vi "SerialRX.vi"() -> ()   [LabVIEW 2015]
uses:
  <vilib>/Instr/_visa.llb/VISA Set IO Buffer Mask.ctl
  <vilib>/Instr/_visa.llb/VISA Configure Serial Port (Instr).vi
  <vilib>/express/express analysis/Spectral/Block/exnSpectralBlock spectral measurements peak poly.vi
  <vilib>/express/express analysis/Spectral/Block/exnSpectralBlock spectral measurements peak DDT.vi
  <vilib>/express/express analysis/Spectral/XNode/ExpressSpectralMeasurementsBlockNode.xnode
  <instrlib>/Siglent SDG 1000 5000 800 Series/Siglent SDG 1000 5000 800 Series.lvlib
panel:
  in  "Boolean":bool
  out "ENOB (db)":dbl
  out "Waveform Graph 4":dbl[](graph)
  out "SINAD (dB)":dbl
  out "Waveform Graph":dynamicdata(graph)
  in  "Waveform Function (0: Sine)":u16(ring) items=["Sine", "Square", "Ramp", "DC", "Pulse", "Arb"]
  in  "Enable Output":bool
  in  "Amplitud ( Vpp )":dbl
  in  "DC Offset ( V )":dbl
  out "THD":dbl
  out "Waveform Graph 3":dynamicdata(graph)
  in  "Serial Settings":T1={"baud rate"=9600, "data bits"=8, "parity"=enum."None", "stop bits"=10, "flow control"=0} {"flow control" items=["None"=0, "XON/XOFF"=1, "RTS/CTS"=2, "DTR/DSR"=4]; "stop bits" items=["1.0"=10, "1.5"=15, "2.0"=20]; "data bits" min=5 max=8 step=1; "baud rate" items=["75"=75, "110"=110, "134"=134, "150"=150, "300"=300, "600"=600, "1200"=1200, "1800"=1800, "2400"=2400, "4800"=4800, "7200"=7200, "9600"=9600, "14400"=14400, "19200"=19200, "28800"=28800, "38400"=38400, "56000"=56000, "57600"=57600, "115200"=115200, "128000"=128000, "230400"=230400]}
  out "Waveform Graph 2":dbl[](graph)
  in  "GENERADOR":refnum<visa-resource-name>
  in  "FPGA":refnum<visa-resource-name>
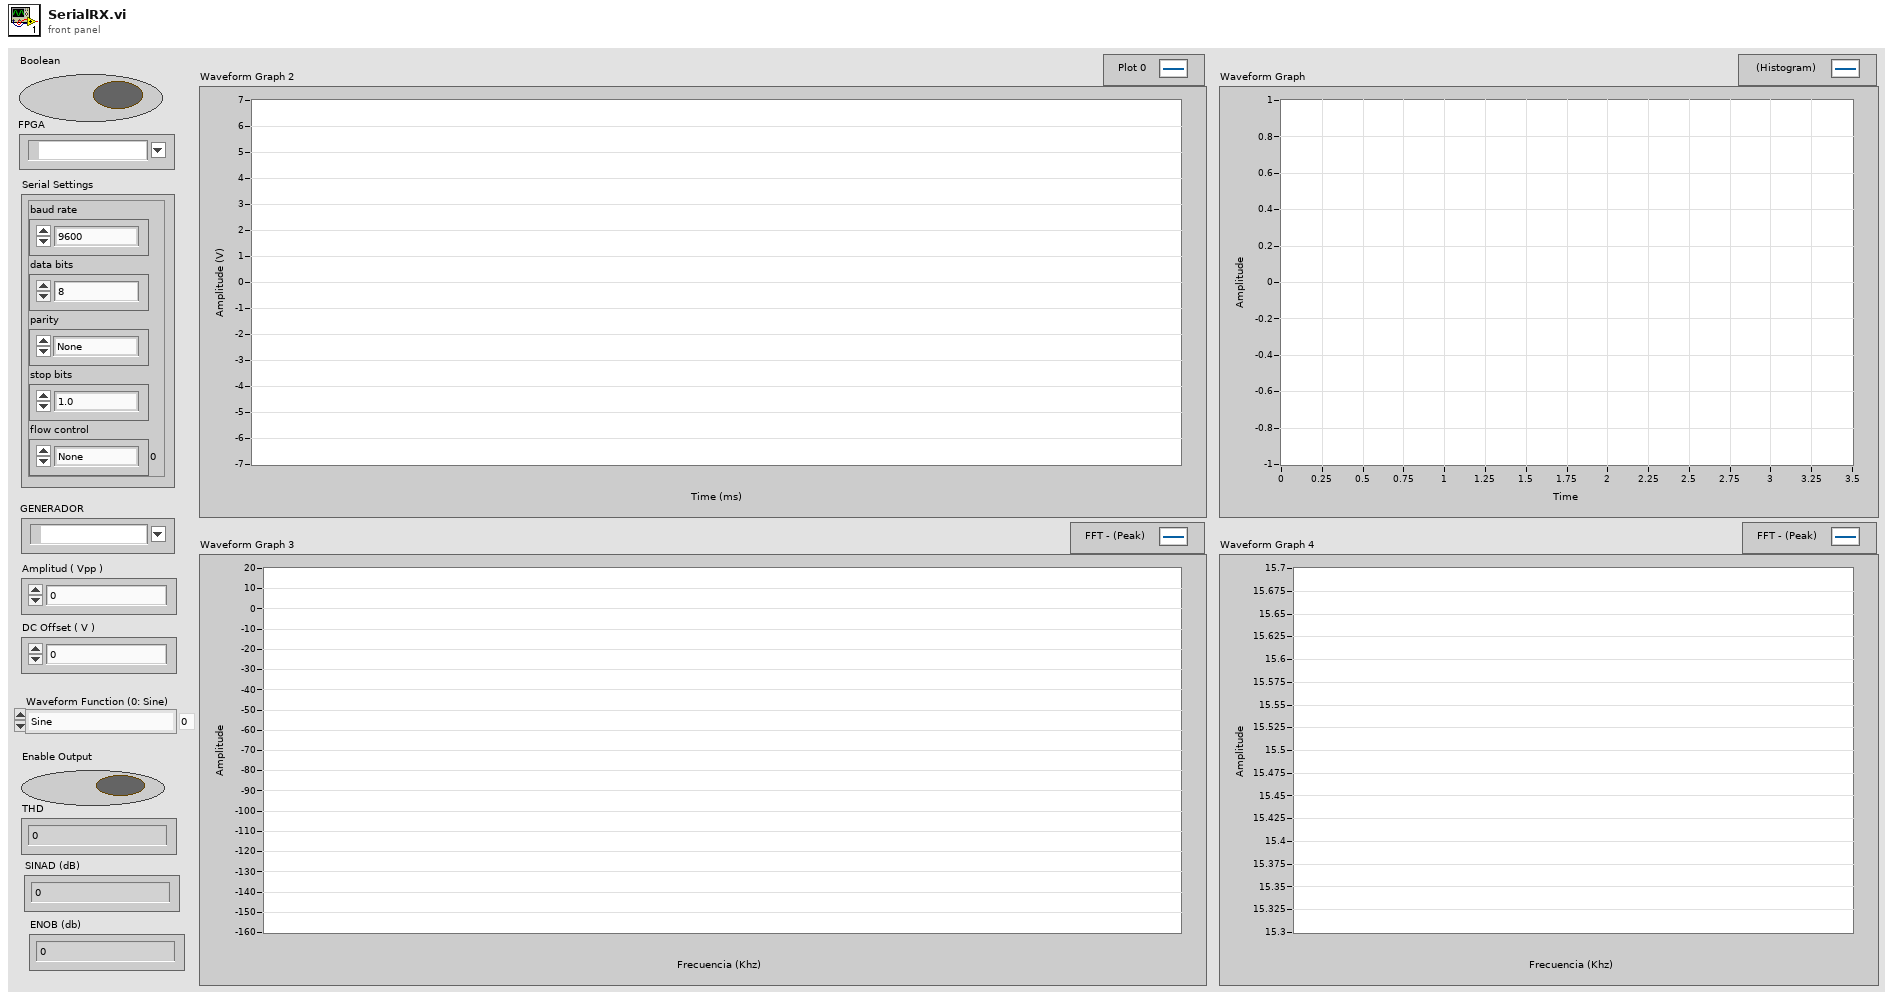
[diagram p1: front panel]
types:
  T1 = cluster{"baud rate":u32, "data bits":u16, "parity":enum16{"None", "Odd", "Even", "Mark", "Space"}, "stop bits":u16, "flow control":u16}
  T2 = typedef "VISA Set IO Buffer Mask.ctl" = u16
  T3 = cluster{"averaging mode":u16, "weighting mode":u16, "number of averages":u32}
  T4 = cluster{"dB On (F)":bool, "unwrap phase (F)":bool, "convert to degree (F)":bool}
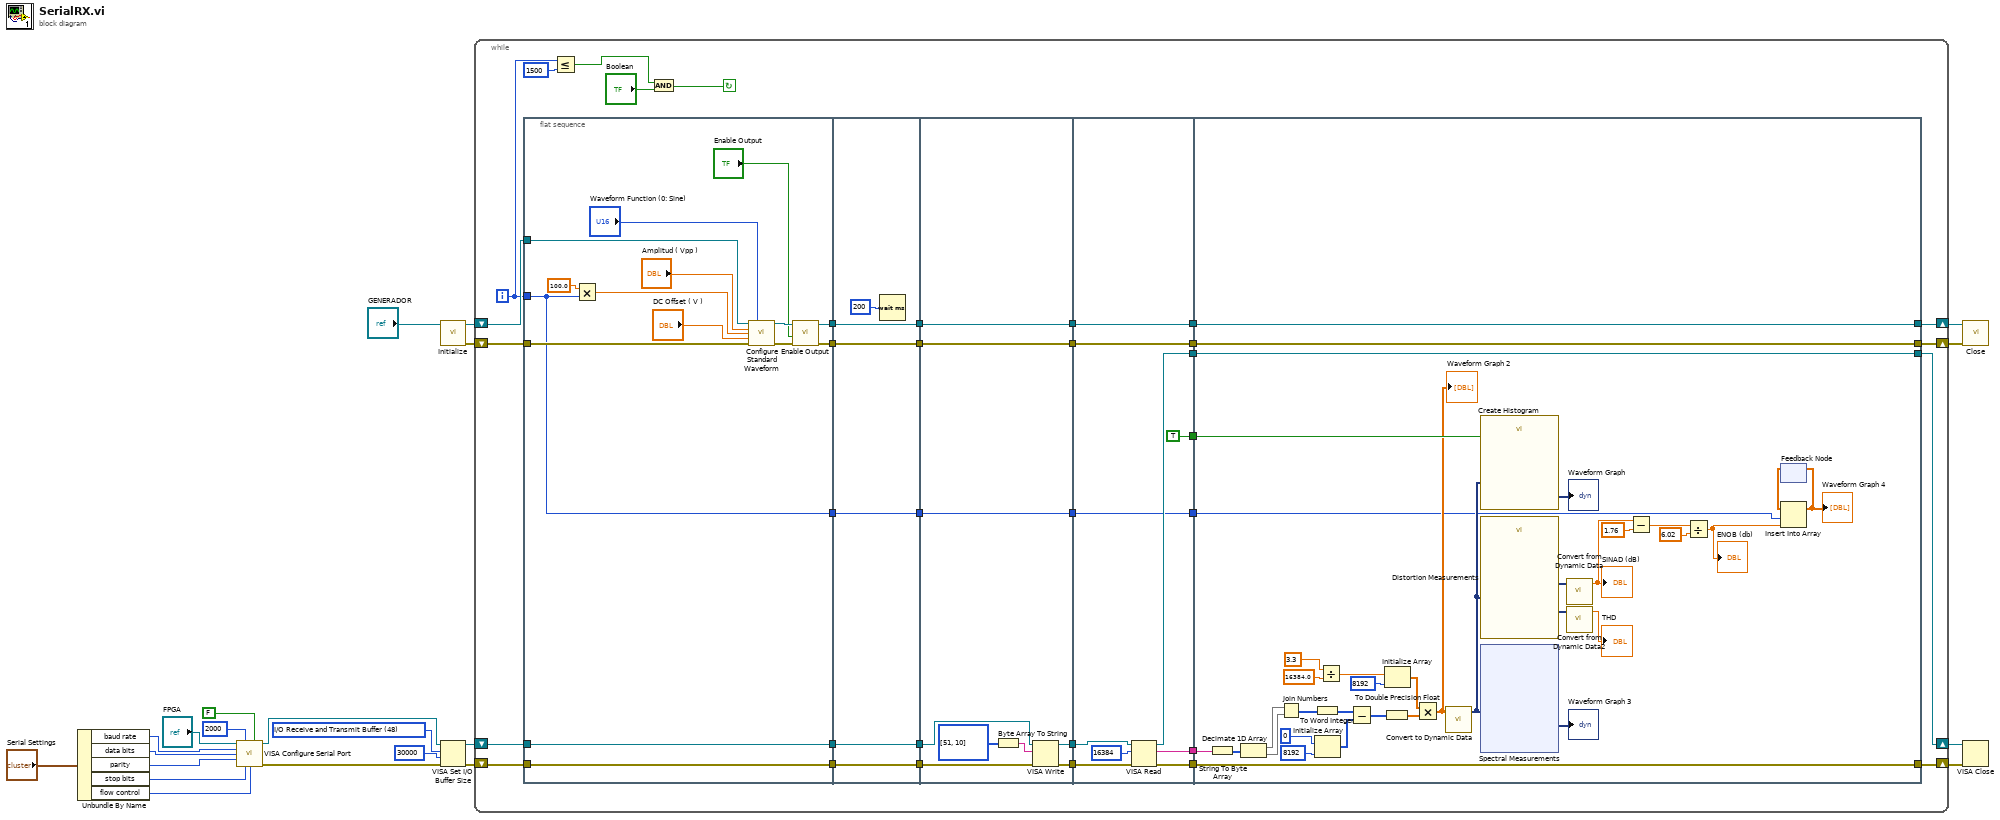
[diagram p0: block diagram]
diagram:
  w1 = T2 48 items=["I/O Receive Buffer"=16, "I/O Transmit Buffer"=32, "I/O Receive and Transmit Buffer"=48] ("Mask")
  n1 = Unbundle By Name("Serial Settings") -> ("baud rate"=w13:u32, "data bits"=w12:u16, "parity"=w11:enum16{"None", "Odd", "Even", "Mark", "Space"}, "stop bits"=w10:u16, "flow control"=w9:u16)
  n2 = call-poly "VISA Configure Serial Port"("VISA resource name"="FPGA", "timeout (10sec)"=u32 2000, "Enable Termination\nChar (T)"=FALSE ("Enable Termination\nChar (T)"), "baud rate (9600)"=w13, "data bits (8)"=w12, "parity (0:none)"=w11, "stop bits (10: 1 bit)"=w10, "flow control (0:none)"=w9) -> ("VISA resource name out"=w4:refnum<visa-resource-name>, "error out"=w3:errorcluster)  [unwired: 6 in]
  n3 = call <instrlib>:"Initialize.vi"("VISA resource name"="GENERADOR") -> ("error out"=w17:errorcluster, "VISA resource name out"=w18:refnum<visa-resource-name>)  [unwired: 9 in]
  n4 = VISA Set I/O Buffer Size(VISA resource name=w4, mask (16)=w1, size (4096)=u32 30000, error in (no error)=w3) -> (VISA resource name out=w6:refnum<visa-resource-name>, error out=w5:errorcluster)
  n5 = while {
    shift-right: [w45] -> w19
    shift-left: w6 -> [w44]
    shift-right: [w46] -> w20
    shift-left: w5 -> [w43]
    shift-right: [w48] -> w22
    shift-left: w18 -> [w42]
    shift-right: [w47] -> w21
    shift-left: w17 -> [w41]
    i -> [w25]
    stop <- w27 continue-if-true
    n6 = flat-sequence {
      tunnel: w42 -> [w70]
      tunnel: w41 -> [w69]
      tunnel: [w66] -> w40
      tunnel: [w68] -> w38
      tunnel: [w67] -> w36
      tunnel: w44 -> [w66]
      tunnel: w43 -> [w65]
      tunnel: [w65] -> w34
      tunnel: w25 -> [w58]
      tunnel: [w58] -> w31
      tunnel: w40 -> [w78]
      tunnel: [w78] -> w39
      tunnel: w38 -> [w77]
      tunnel: [w77] -> w37
      tunnel: w36 -> [w76]
      tunnel: [w76] -> w35
      tunnel: w34 -> [w75]
      tunnel: [w75] -> w33
      tunnel: w31 -> [w73]
      tunnel: [w73] -> w30
      tunnel: w39 -> [w87]
      tunnel: [w85] -> w57
      tunnel: [w84] -> w56
      tunnel: w37 -> [w83]
      tunnel: [w83] -> w55
      tunnel: w35 -> [w82]
      tunnel: [w82] -> w54
      tunnel: w33 -> [w86]
      tunnel: w30 -> [w79]
      tunnel: [w79] -> w29
      tunnel: w57 -> [w97]
      tunnel: w56 -> [w96]
      tunnel: [w94] -> w53
      tunnel: w55 -> [w93]
      tunnel: [w93] -> w52
      tunnel: w54 -> [w92]
      tunnel: [w92] -> w51
      tunnel: [w91] -> w50
      tunnel: [w90] -> w49
      tunnel: [TRUE] -> w32
      tunnel: w29 -> [w88]
      tunnel: [w88] -> w28
      tunnel: w53 -> [w131]
      tunnel: w52 -> [w133]
      tunnel: w51 -> [w132]
      tunnel: w50 -> [w128]
      tunnel: w49 -> [w129]
      tunnel: [w133] -> w48
      tunnel: [w132] -> w47
      tunnel: [w128] -> w45
      tunnel: [w129] -> w46
      tunnel: w32 -> [w113]
      tunnel: w28 -> [w105]
      frame #0 {
        n7 = Multiply(x=100.0, y=w58) -> (x*y=w59:dbl)
        n8 = call <instrlib>:"Configure Standard Waveform.vi"("VISA resource name"=w70, "Waveform Function (0: Sine)"="Waveform Function (0: Sine)", "Amplitude (1.0 Vpp)"="Amplitud ( Vpp )", "Frequency (1000 Hz)"=w59, "DC Offset (0.00 V)"="DC Offset ( V )", "error in (no error)"=w69) -> ("VISA resource name out"=w72:refnum<visa-resource-name>, "error out"=w71:errorcluster)  [unwired: 8 in]
        n9 = call <instrlib>:"Enable Output.vi"("error in (no error)"=w71, "Enable Output (T: Enable)"="Enable Output", "VISA resource name"=w72) -> ("error out"=w67:errorcluster, "VISA resource name out"=w68:refnum<visa-resource-name>)  [unwired: 7 in]
      }
      frame #1 {
        n10 = Wait (ms)(milliseconds to wait=u32 200) -> ()  [unwired: 1 out]
      }
      frame #2 {
        n11 = Byte Array To String(unsigned byte array=u8[] [51, 10]) -> (string=w80:string)
        n12 = VISA Write(VISA resource name=w87, write buffer=w80, error in (no error)=w86) -> (VISA resource name out=w85:refnum<visa-resource-name>, error out=w84:errorcluster)  [unwired: 1 out]
      }
      frame #3 {
        n13 = VISA Read(VISA resource name=w97, byte count=u32 16384, error in (no error)=w96) -> (VISA resource name out=w91:refnum<visa-resource-name>, read buffer=w94:string, error out=w90:errorcluster)  [unwired: 1 out]
      }
      frame #4 {
        n14 = String To Byte Array(string=w131) -> (unsigned byte array=w130:u8[])
        n15 = Decimate 1D Array(w130) -> (w126:u8[], w125:u8[])
        n16 = Join Numbers(hi=w126, lo=w125) -> ((hi.lo)=w99:u16[])
        n17 = To Word Integer(number=w99) -> (16bit integer=w98:i16[])
        n18 = Initialize Array(i16 0 ("element"), 8192 ("dimension size")) -> (w120:i16[])
        n19 = Divide(x=3.3, y=16384.0) -> (x/y=w119:dbl)
        n20 = Subtract(x=w98, y=w120) -> (x-y=w116:i16[])
        n21 = Initialize Array(w119, 8192 ("dimension size")) -> (w123:dbl[])
        n22 = To Double Precision Float(number=w116) -> (double precision float=w115:dbl[])
        n23 = Multiply(x=w123, y=w115) -> (x*y=w112:dbl[])
        "Waveform Graph 2" <- w112
        n24 = call "Convert to Dynamic Data"("Array"=w112) -> ("Dynamic Data Type"=w110:dynamicdata)  [unwired: 3 in]
        n25 = call "Create Histogram"("Reset"=w113, "Signal"=w110) -> ("Histogram"=→"Waveform Graph":dynamicdata)  [unwired: 8 in, 1 out]
        n26 = call "Distortion Measurements"("Signals"=w110) -> ("SINAD (dB)"=w109:dynamicdata, "THD"=w107:dynamicdata)  [unwired: 7 in, 2 out]
        n27 = xnode "Spectral Measurements"("Signals"=w110) -> ("FFT - (Peak)"=→"Waveform Graph 3":dynamicdata)  [unwired: 1 in, 2 out]
        n28 = call "Convert from Dynamic Data"("Dynamic Data Type"=w109) -> ("Scalar"=w104:dbl)  [unwired: 3 in]
        "SINAD (dB)" <- w104
        n29 = call "Convert from Dynamic Data2"("Dynamic Data Type"=w107) -> ("Scalar"=→"THD":dbl)  [unwired: 3 in]
        n30 = Subtract(x=w104, y=1.76) -> (x-y=w102:dbl)
        n31 = Divide(x=w102, y=6.02) -> (x/y=w100:dbl)
        "ENOB (db)" <- w100
        n32 = feedback #1() -> (w111:dbl[])  [unwired: 1 in]
        n33 = Insert Into Array(array=w111, index=w105, new element=w100) -> (w106:dbl[])
        "Waveform Graph 4" <- w106
        n34 = feedback-in #1(w106) -> ()
      }
    }
    n35 = Less Or Equal?(x=w25, y=1500) -> (x <= y?=w23:bool)
    n36 = And(x=w23, y="Boolean") -> (x .and. y?=w27:bool)
  }
  n37 = call <instrlib>:"Close.vi"("error in (no error)"=w21, "VISA resource name"=w22) -> ()  [unwired: 9 in, 1 out]
  n38 = VISA Close(VISA resource name=w19, error in (no error)=w20) -> ()  [unwired: 1 out]
